vi "SLAM_emulation.vi"(7 "X":dbl[](array[numeric]), 8 "error in":errorcluster, 9 "measurements":dbl[][](array[numeric]), 10 "dX":dbl[](array[numeric]), 11 "P":dbl[][](array[numeric])) -> (0 "error out":errorcluster, 1 "measuredLandmarks":dbl[][](array[numeric]), 2 "Xodometry":dbl[](array[numeric]), 3 "Pout":dbl[][](array[numeric]), 5 "Xout":dbl[](array[numeric]))   [LabVIEW 2009, in "Main.lvlib"]
uses:
  Main.lvlib
  Drive/Drive_Utils.lvlib
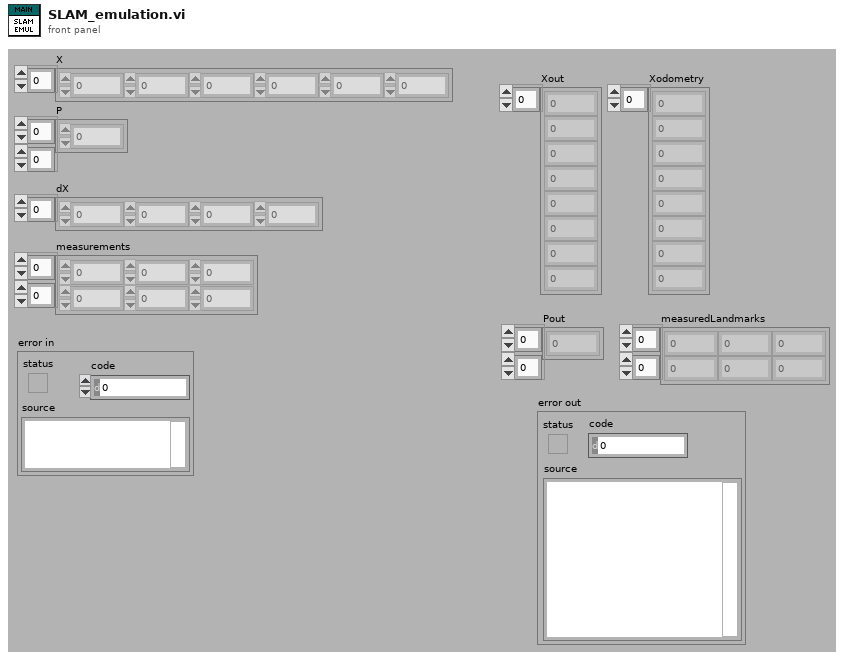
[diagram p1: front panel]
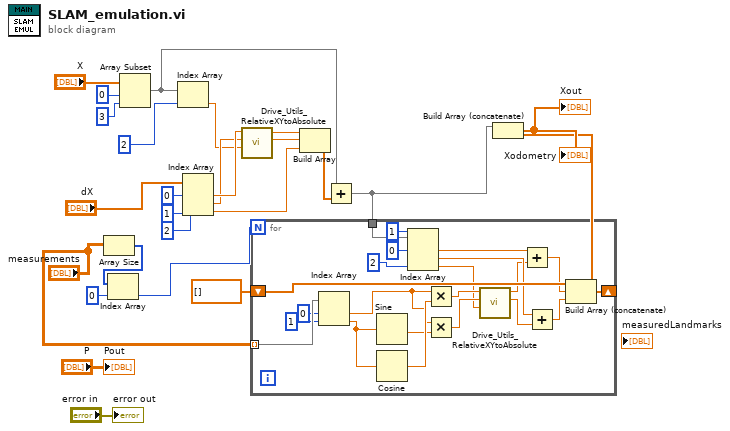
[diagram p0: block diagram]
diagram:
  n1 = Array Size(array="measurements") -> (size(s)=w8:i32[])
  n2 = Index Array(array=w8, index=0) -> (element=w5:i32)
  n3 = Array Subset(array="X", index=0, length=3) -> (w10:dbl[])
  n4 = Index Array(array=w10, index=2) -> (element=w4:dbl)
  n5 = Index Array(array="dX", index #1=0 ("index"), index #2=1 ("index"), index #3=2 ("index")) -> (element #1=w17:dbl, element #2=w16:dbl, element #3=w14:dbl)
  n6 = call "Drive_Utils_RelativeXYtoAbsolute.vi"("Angle"=w4, "Y"=w16, "X"=w17) -> ("Y"=w13:dbl, "X"=w12:dbl)  [unwired: 2 in, 1 out]
  n7 = Build Array(w12, w13, w14) -> (w11:dbl[])
  n8 = Add(x=w10, y=w11) -> (x+y=w1:dbl[])
  n9 = for {
    N: w5 -> [_]
    tunnel: "measurements" -> [w48] mode=indexing
    shift-right: [w39] -> w2
    shift-left: dbl[] [] -> [w38]
    tunnel: w1 -> [w37]
    n10 = Index Array(array=w48, index #1=0 ("index"), index #2=1 ("index")) -> (element #1=w42:dbl, element #2=w45:dbl)
    n11 = Sine(x=w45) -> (sin(x)=w41:dbl)
    n12 = Cosine(x=w45) -> (cos(x)=w44:dbl)
    n13 = Index Array(array=w37, index #1=0 ("index"), index #2=1 ("index"), index #3=2 ("index")) -> (element #1=w32:dbl, element #2=w31:dbl, element #3=w35:dbl)
    n14 = Multiply(x=w42, y=w44) -> (x*y=w43:dbl)
    n15 = Multiply(x=w42, y=w41) -> (x*y=w40:dbl)
    n16 = call "Drive_Utils_RelativeXYtoAbsolute.vi"("Angle"=w35, "Y"=w40, "X"=w43) -> ("Y"=w28:dbl, "X"=w30:dbl)  [unwired: 2 in, 1 out]
    n17 = Add(x=w32, y=w30) -> (x+y=w29:dbl)
    n18 = Add(x=w31, y=w28) -> (x+y=w27:dbl)
    n19 = Build Array (concatenate)(w38, w29, w27) -> (w39:dbl[])
  }
  n20 = Build Array (concatenate)(w1, w2) -> (→"Xout" →"Xodometry":dbl[])
  "Pout" <- "P"
  "error out" <- "error in"
